vi "finalize digestsign.vi"(8 "error in":errorcluster, 11 "lvlibcrypto digest in":refnum<class "lvlibcrypto digestsign.lvclass">) -> (0 "error out":errorcluster, 3 "digest":string)   [LabVIEW 2016, in "lvlibcrypto digestsign.lvclass"]
uses:
  lvlibcrypto digestsign.lvclass
  lvlibcrypto digestsign.lvclass/lvlibcrypto digestsign.ctl
  lv tls dll.lvlib
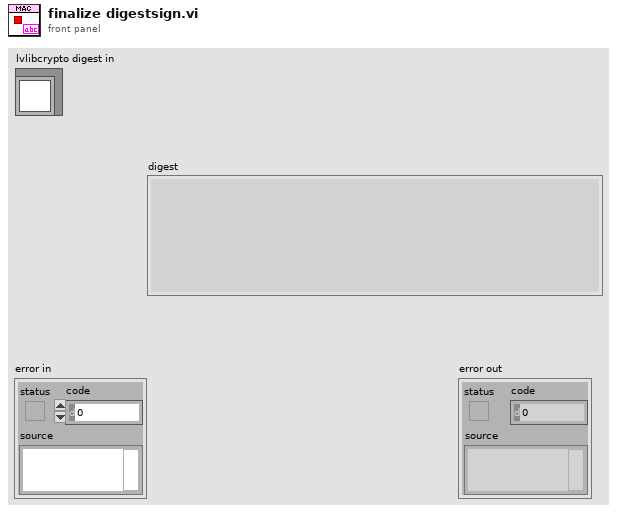
[diagram p1: front panel]
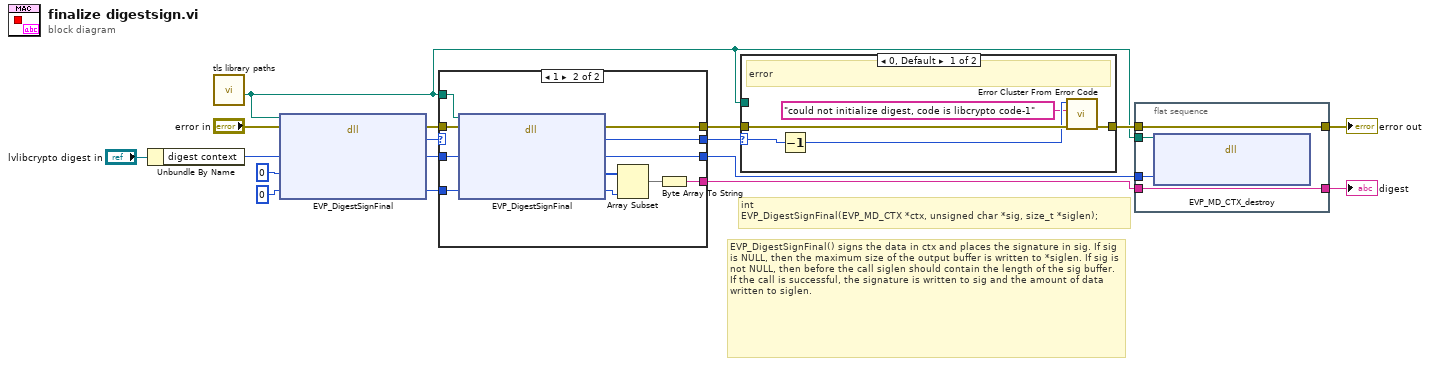
[diagram p0: block diagram]
diagram:
  # "EVP_DigestSignFinal() signs the data in ctx and places the signature in sig. If sig is NULL, then the maximum size of the output buffer is written to *siglen. If sig is not NULL, then before the call siglen should contain the length of the sig buffer. If the call is successful, the signature is written to sig and the amount of data written to siglen."
  # "int \nEVP_DigestSignFinal(EVP_MD_CTX *ctx, unsigned char *sig, size_t *siglen);"
  n1 = Unbundle By Name("lvlibcrypto digest in") -> ("digest context"=w11:u64)
  n2 = call "tls library paths.vi"() -> ("libcrypto"=w1:path)  [unwired: 8 in, 3 out]
  n3 = dll-call lib="C:/Users/IEUser/Desktop/tlssimple/libcrypto-41.dll" fn="EVP_DigestSignFinal"(path in=w1, error in="error in", "context"=w11, "digest"=u64 0, "length"=u32 0) -> (error out=w12:errorcluster, "ret"=w2:i32, "context"=w3:u64, "length"=w8:u32)  [unwired: 2 in, 1 out]
  n4 = case shown="1" w2 {
    selector: w2 -> [w18 _]
    tunnel: [w18 w31] -> w16
    tunnel: [w19 w30] -> w15
    tunnel: [w20 w29] -> w14
    tunnel: w1 -> [_ w25]
    tunnel: w12 -> [w19 w24]
    tunnel: w8 -> [_ w23]
    tunnel: [_ w22] -> w5
    tunnel: w3 -> [w20 w21]
    frame 0, Default {
    }
    frame 1 {
      n5 = dll-call lib="C:/Users/IEUser/Desktop/tlssimple/libcrypto-41.dll" fn="EVP_DigestSignFinal"(path in=w25, error in=w24, "context"=w21, "length"=w23) -> (error out=w30:errorcluster, "ret"=w31:i32, "context"=w29:u64, "digest"=w28:u8[], "length"=w27:u32)  [unwired: 2 in, 1 out]
      n6 = Array Subset(array=w28, length=w27) -> (w26:u8[])  [unwired: 1 in]
      n7 = Byte Array To String(unsigned byte array=w26) -> (string=w22:string)
    }
  }
  n8 = case shown="0, Default" w16 {
    selector: w16 -> [w34 _]
    tunnel: [w35 w37] -> w7
    tunnel: w15 -> [w36 w37]
    tunnel: w1 -> [_ _]
    frame 0, Default {
      # "error"
      n9 = Decrement(x=w34) -> (x-1=w33:i32)
      n10 = call <vilib>:"Error Cluster From Error Code.vi"("error in (no error)"=w36, "error message (\"\")"="could not initialize digest, code is libcrypto code-1" ("error message (\"\")"), "error code (0)"=w33) -> ("error out"=w35:errorcluster)  [unwired: 6 in]
    }
    frame 1 {
      # "success"
    }
  }
  n11 = flat-sequence {
    tunnel: w1 -> [w41]
    tunnel: w14 -> [w40]
    tunnel: [w39] -> w6
    tunnel: w7 -> [w39]
    tunnel: w5 -> [w38]
    tunnel: [w38] -> w4
    frame #0 {
      n12 = dll-call lib="C:/Users/IEUser/Desktop/tlssimple/libcrypto-41.dll" fn="EVP_MD_CTX_destroy"(path in=w41, "context"=w40) -> ()  [unwired: 4 in, 2 out]
    }
  }
  "error out" <- w6
  "digest" <- w4
